vi "Agilent 34970 Matrix Switch.vi"() -> ()   [LabVIEW 2015]
doc: "This VI shows you how to use the HP34904A Matrix Switch.\n\nFirst, select the crosspoint(s) you wish to close. Do this by pressing down the button(s) corresponding to the desired crosspoint(s). Then, press the run button on the LabVIEW toolbar.\n\nAny crosspoint whose button is not pressed down will be opened."
uses:
  Agilent 34970.lvlib
panel:
  in  "Serial Port Configuration":T1={"Timeout Value (10000)"=10000, "Baud Rate (57600)"=enum."57600", "Flow Control (1:XON/XOFF)"=enum."XON / XOFF"}
  in  "Reset (T: Reset)":bool=TRUE
  in  "VISA resource name":refnum<visa-resource-name>
  in  "Cross Points (F = open)":bool[][](array[boolean])=[[FALSE, FALSE, FALSE, FALSE, FALSE, FALSE, FALSE, FALSE], [FALSE, FALSE, FALSE, FALSE, FALSE, FALSE, FALSE, FALSE], [FALSE, FALSE, FALSE, FALSE, FALSE, FALSE, FALSE, FALSE], [FALSE, FALSE, FALSE, FALSE, FALSE, FALSE, FALSE, FALSE]]
  in  "Slot Number":u8=1 min=1 max=3 step=1
  # "(c) 2005-2010 National Instruments.  ALL RIGHTS RESERVED."
  # "This Example VI demonstrates using the matrix switching abilities of the HP34970A.  The 34904A is organized in a 4x8 grid that can be controlled using the LEDs above.  Setting a LED to off (False) will open the crosspoint.\n\nUse the Slot Number control to choose which of the three module  slots to access."
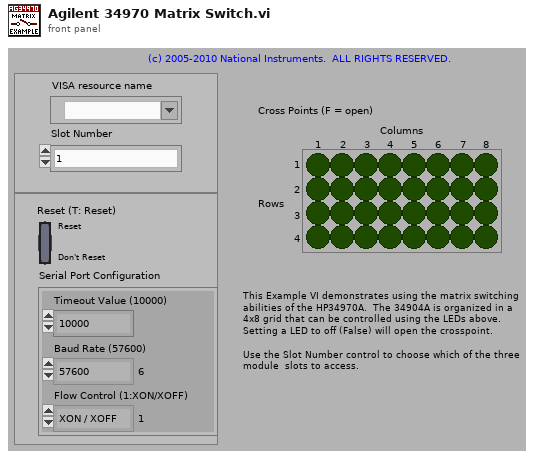
[diagram p1: front panel]
types:
  T1 = cluster{"Timeout Value (10000)":u32, "Baud Rate (57600)":enum16{"1200", "2400", "4800", "9600", "19200", "38400", "57600", "115200"}, "Flow Control (1:XON/XOFF)":enum16{"None", "XON / XOFF", "RTS / CTS", "DTR / DSR"}}
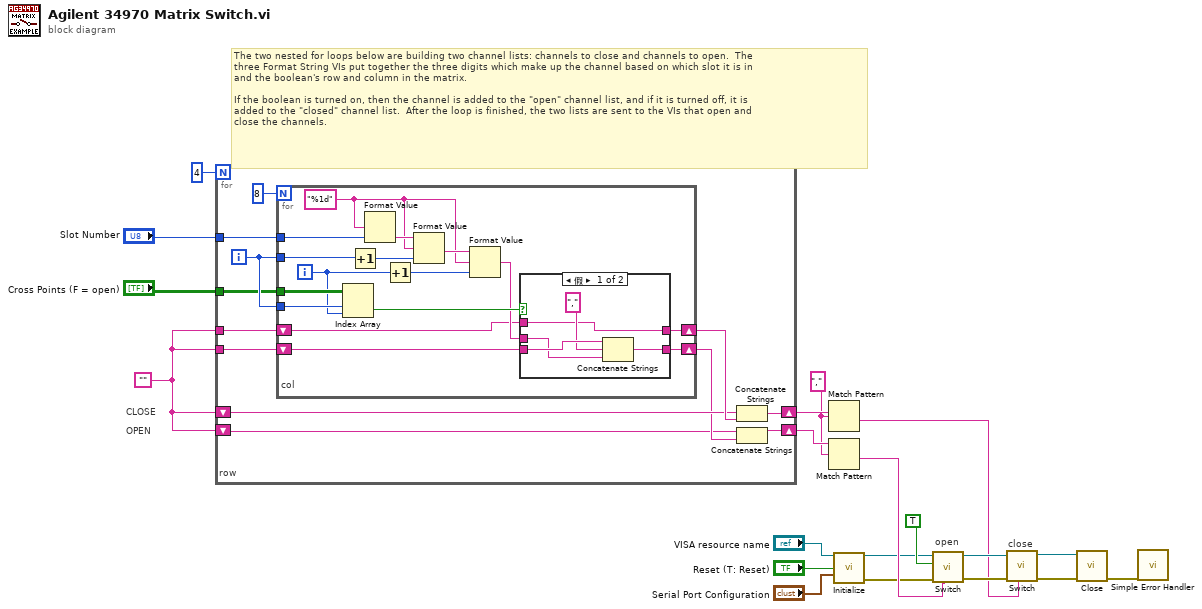
[diagram p0: block diagram]
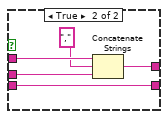
[diagram p2: hidden frame]
diagram:
  w15 = "," ("output string")
  w18 = "" ("Empty String Constant")
  # "The two nested for loops below are building two channel lists: channels to close and channels to open.  The \nthree Format String VIs put together the three digits which make up the channel based on which slot it is in\nand the boolean's row and column in the matrix.\n\nIf the boolean is turned on, then the channel is added to the \"open\" channel list, and if it is turned off, it is\nadded to the \"closed\" channel list.  After the loop is finished, the two lists are sent to the VIs that open and \nclose the channels."
  # "close"
  # "open"
  # "OPEN"
  # "CLOSE"
  n1 = for {
    N: u16 4 ("y") -> [_]
    tunnel: "Slot Number" -> [w32]
    shift-right: [w24] -> w17
    shift-left: w18 -> [w25]
    shift-right: [w23] -> w16
    shift-left: w18 -> [w21]
    tunnel: "Cross Points (F = open)" -> [w30]
    tunnel: w18 -> [w28]
    tunnel: w18 -> [w27]
    i -> [w31]
    # "row"
    n2 = for {
      N: u16 8 ("y") -> [_]
      tunnel: w31 -> [w48]
      tunnel: w32 -> [w47]
      tunnel: w31 -> [w37]
      tunnel: w30 -> [w44]
      shift-right: [w40] -> w26
      shift-left: w28 -> [w41]
      shift-right: [w38] -> w22
      shift-left: w27 -> [w39]
      i -> [w34]
      w33 = "%1d" ("format string")
      # "col"
      n3 = Index Array(array=w44, index (row)=w48, index (col)=w34) -> (element=w43:bool)
      n4 = Increment(x=w37) -> (x+1=w36:i32)
      n5 = Format Value(format string=w33, value (0)=w47) -> (output string=w46:string)  [unwired: 1 in]
      n6 = Increment(x=w34) -> (x+1=w35:i32)
      n7 = Format Value(string ("")=w46, format string=w33, value (0)=w36) -> (output string=w45:string)
      n8 = Format Value(string ("")=w45, format string=w33, value (0)=w35) -> (output string=w42:string)
      n9 = case shown="假" w43 {
        tunnel: w42 -> [w49 w56]
        tunnel: w41 -> [w50 w58]
        tunnel: [w50 w57] -> w40
        tunnel: w39 -> [w53 w54]
        tunnel: [w52 w54] -> w38
        frame False {
          n10 = Concatenate Strings(w53, "," ("output string"), w49) -> (w52:string)
        }
        frame True {
          n11 = Concatenate Strings(w58, "," ("output string"), w56) -> (w57:string)
        }
      }
    }
    n12 = Concatenate Strings(w25, w26) -> (w24:string)
    n13 = Concatenate Strings(w21, w22) -> (w23:string)
  }
  n14 = Match Pattern(string=w17, regular expression=w15) -> (after substring=w10:string)  [unwired: 1 in, 3 out]
  n15 = Match Pattern(string=w16, regular expression=w15) -> (after substring=w13:string)  [unwired: 1 in, 3 out]
  n16 = call <instrlib>:"Initialize.vi"("VISA Resource Name"="VISA resource name", "Reset (T: Reset)"="Reset (T: Reset)", "Serial Port Configuration"="Serial Port Configuration") -> ("VISA Resource Name Out"=w8:refnum<visa-resource-name>, "error out"=w7:errorcluster)  [unwired: 11 in]
  n17 = call <instrlib>:"Switch.vi"("Channel List(empty)"=w13, "error in (no error)"=w7, "Open/Close (F:Close)"=TRUE ("Open/Close"), "VISA Resource Name"=w8) -> ("error out"=w12:errorcluster, "VISA Resource Name Out"=w11:refnum<visa-resource-name>)  [unwired: 5 in, 1 out]
  n18 = call <instrlib>:"Switch.vi"("Channel List(empty)"=w10, "error in (no error)"=w12, "VISA Resource Name"=w11) -> ("error out"=w2:errorcluster, "VISA Resource Name Out"=w3:refnum<visa-resource-name>)  [unwired: 6 in, 1 out]
  n19 = call <instrlib>:"Close.vi"("VISA Resource Name"=w3, "error in (no error)"=w2) -> ("error out"=w1:errorcluster)  [unwired: 13 in]
  n20 = call <vilib>:"Simple Error Handler.vi"("error in (no error)"=w1) -> ()  [unwired: 4 in, 5 out]
